vi "Paths.vi"(7 "PNG file path":path) -> (3 "Traces.txt path":path, 4 "Pixmap.bin path":path, 6 "Extract path":path, 8 "VI folder":path, 10 "PDF file path":path, 13 "Paths error":errorcluster, 14 "PNG file name":string, 15 "Script.m path":path)   [LabVIEW 2023]
panel:
  in  "User interface":T1(tab)
  in  "User entries":enum32{""}(tab)
  in  "Customization":enum32{"Customization"}(tab)
  in  "Colors":enum32{"Colors"}(tab)
  in  "Size":enum32{"Size"}(tab)
  in  "Loop FOR 1":enum32{"Loop FOR 1"}(tab)
  in  "Arrays":enum32{"Arrays"}(tab)
  in  "Script.m":enum32{"Script.m"}(tab)
  in  "Extract.c output string scan":enum32{"Extract.c output string scan"}(tab)
  in  "T: tt1 tt2 tt3 ...":enum32{"T: tt1 tt2 tt3 ..."}(tab)
  in  "C: cc":enum32{"C: cc"}(tab)
  in  "Loop FOR 2":enum32{"Loop FOR 2"}(tab)
  in  "LabVIEW":enum32{"LabVIEW"}(tab)
  out "VI's path":path
  in  "MATLAB":enum32{"MATLAB"}(tab)
  out "Script.m file name":string
  in  "C":enum32{"C"}(tab)
  in  "MATLAB":enum32{"MATLAB"}(tab)
  in  "C":enum32{"C"}(tab)
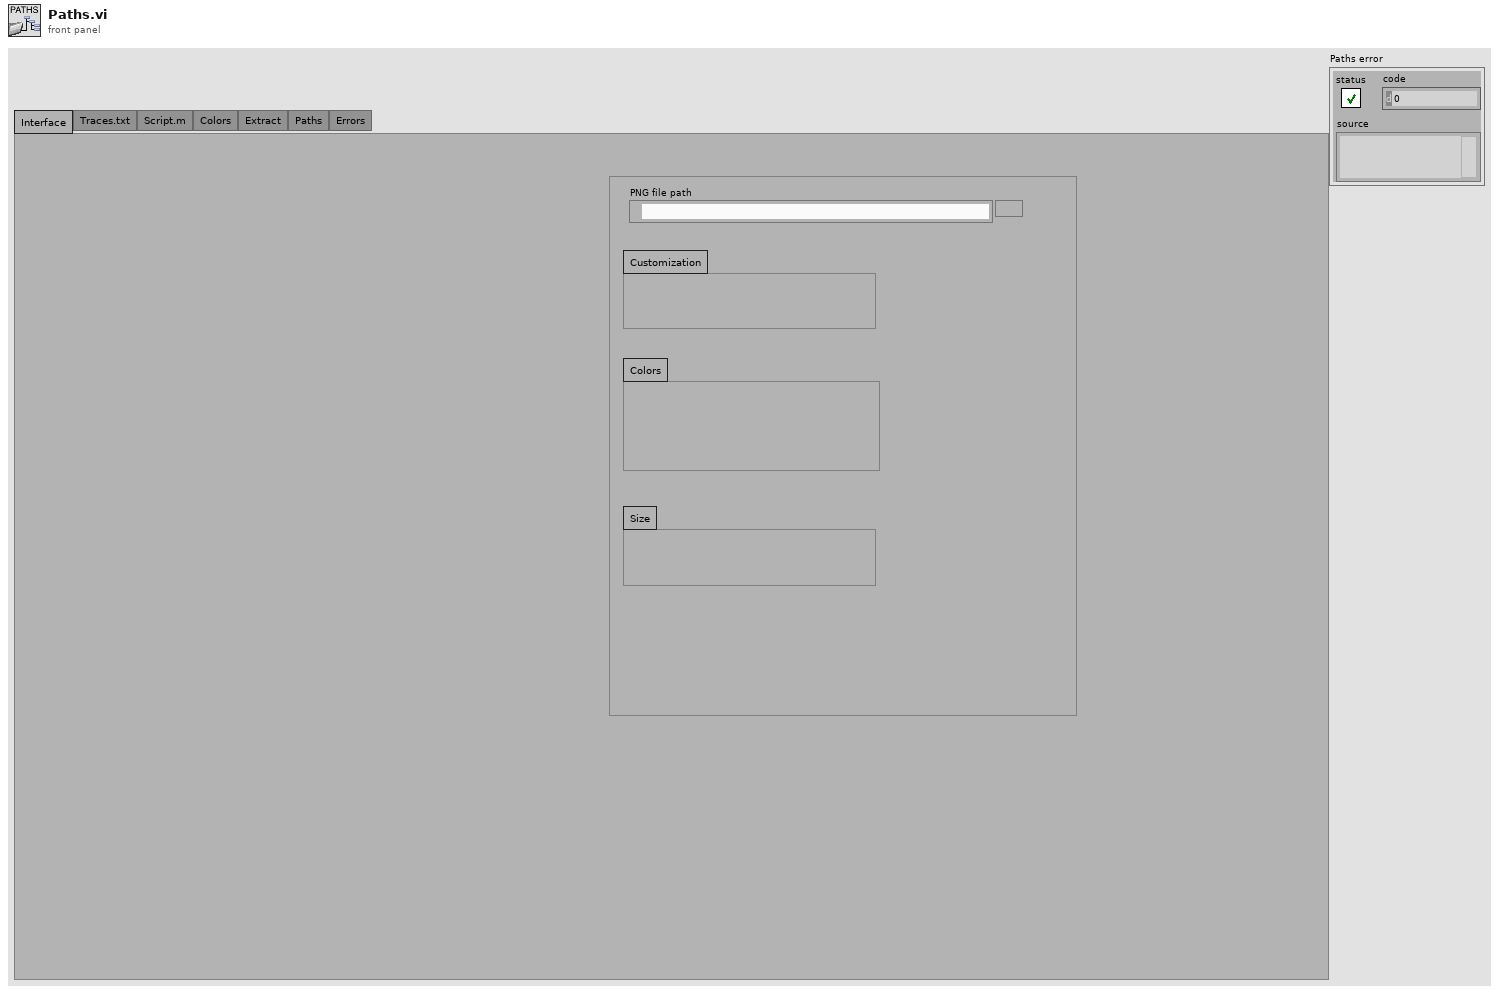
[diagram p1: front panel]
types:
  T1 = enum32{"Interface", "Traces.txt", "Script.m", "Colors", "Extract", "Paths", "Errors"}
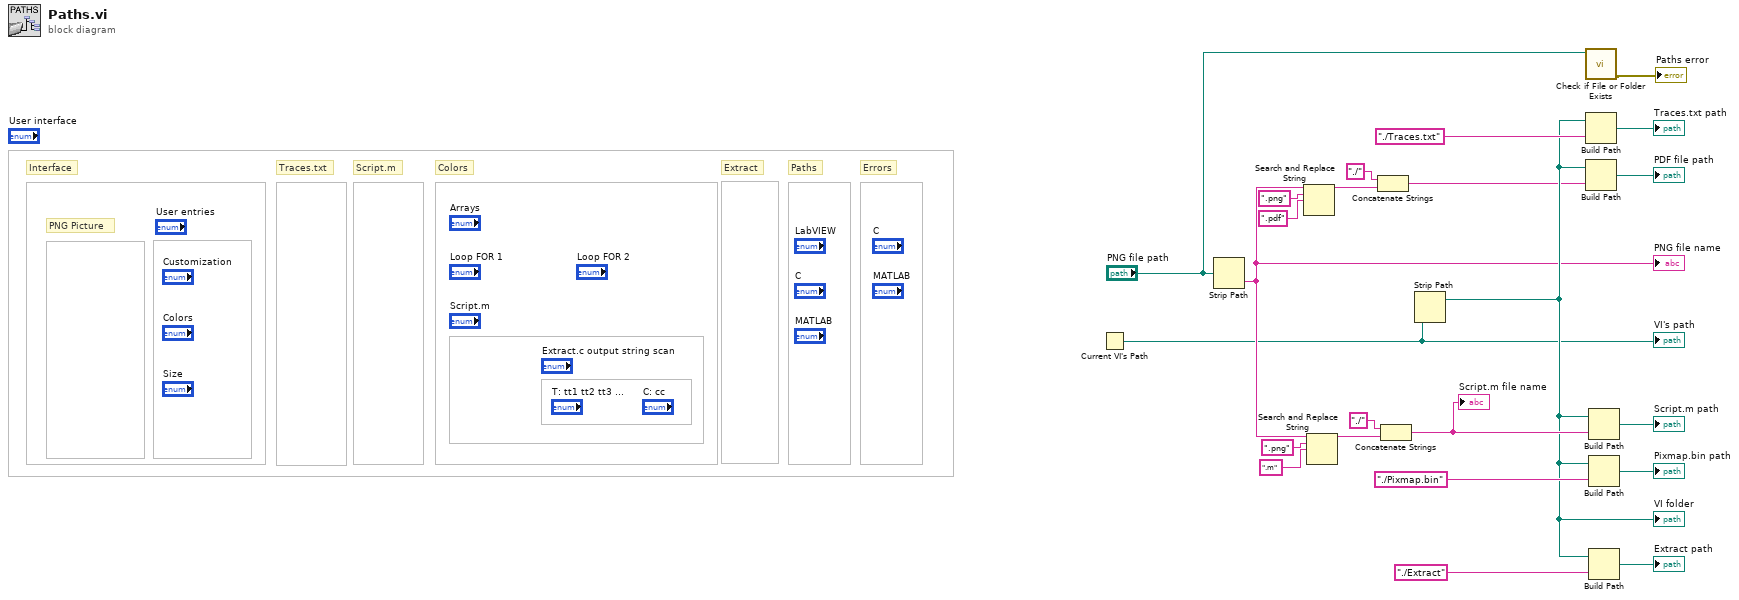
[diagram p0: block diagram]
diagram:
  # "PNG Picture"
  # "Errors"
  # "Paths"
  # "Extract"
  # "Colors"
  # "Script.m"
  # "Traces.txt"
  # "Interface"
  n1 = Current VI's Path() -> (path=w3:path)
  "VI's path" <- w3
  n2 = Strip Path(path="PNG file path") -> (name=w5:string)  [unwired: 1 out]
  "PNG file name" <- w5
  n3 = Search and Replace String(input string=w5, search string=".png", replace string=".pdf" ("replace string (\"\")")) -> (result string=w8:string)  [unwired: 5 in, 3 out]
  n4 = Search and Replace String(input string=w5, search string=".png", replace string=".m" ("replace string (\"\")")) -> (result string=w12:string)  [unwired: 5 in, 3 out]
  n5 = Concatenate Strings("./" ("string"), w8) -> (w6:string)
  n6 = Concatenate Strings("./" ("string"), w12) -> (w14:string)
  "Script.m file name" <- w14
  n7 = Strip Path(path=w3) -> (stripped path=w11:path)  [unwired: 1 out]
  "VI folder" <- w11
  n8 = call <vilib>:"Check if File or Folder Exists.vi"("path"="PNG file path") -> ("error out"=→"Paths error":errorcluster)  [unwired: 8 in, 2 out]
  n9 = Build Path(base path=w11, name or relative path="./Traces.txt") -> (appended path=→"Traces.txt path":path)
  n10 = Build Path(base path=w11, name or relative path=w6) -> (appended path=→"PDF file path":path)
  n11 = Build Path(base path=w11, name or relative path=w14) -> (appended path=→"Script.m path":path)
  n12 = Build Path(base path=w11, name or relative path="./Pixmap.bin") -> (appended path=→"Pixmap.bin path":path)
  n13 = Build Path(base path=w11, name or relative path="./Extract") -> (appended path=→"Extract path":path)
